vi "Insert Stop Message.vi"(8 "error in (no error)":errorcluster, 11 "TimeStamper in":refnum<class "TimeStamper.lvclass">) -> (0 "error out":errorcluster, 3 "TimeStamper out":refnum<class "TimeStamper.lvclass">)   [LabVIEW 2014, in "TimeStamper.lvclass"]
uses:
  TimeStamper.lvclass
  Database/SessionPrimary.ctl
  AcquistionObject/AcquistionObject.lvclass
panel:
  out "resulting string":string
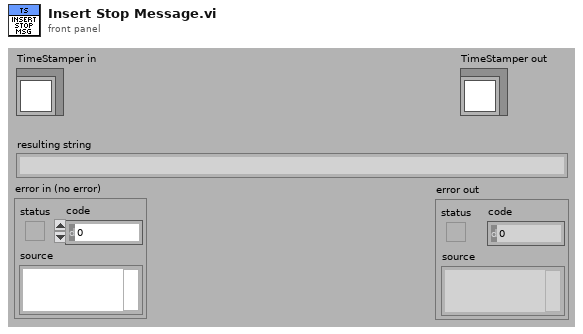
[diagram p1: front panel]
types:
  T1 = typedef "SessionPrimary.ctl" = cluster{"setup":u8, "subject_id":i32, "session_start_time":dbl}
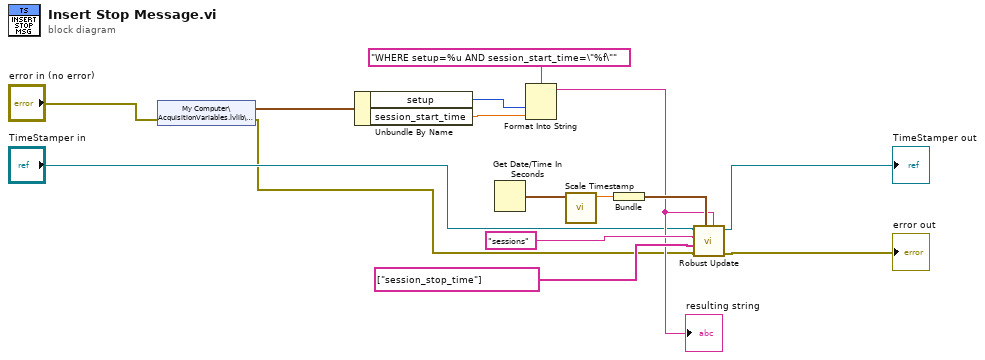
[diagram p0: block diagram]
diagram:
  n1 = shared-variable "My Computer\\AcquisitionVariables.lvlib\\SessionPK"(error in="error in (no error)") -> (w13:T1, error out=w2:errorcluster)
  n2 = Unbundle By Name(w13) -> ("setup"=w11:u8, "session_start_time"=w10:dbl)
  n3 = Get Date/Time In Seconds() -> (seconds since 1Jan1904=w14:timestamp)
  n4 = Format Into String(format string="WHERE setup=%u AND session_start_time=\"%f\"", w11, w10) -> (resulting string=w4:string)  [unwired: 2 in, 1 out]
  "resulting string" <- w4
  n5 = call "Scale Timestamp.vi"("Time Stamp"=w14) -> ("Scaled timestamp"=w9:dbl)  [unwired: 10 in]
  n6 = Bundle("Scaled timestamp"=w9) -> (w5:cluster{"Scaled timestamp":dbl})  [unwired: 1 in]
  n7 = call "Robust Update.vi"("condition"=w4, "data"=w5, "error in (no error)"=w2, "columns"=string[] ["session_stop_time"], "table"="sessions", "AcquistionObject.lvclass"="TimeStamper in") -> ("error out"=→"error out":errorcluster, "AcquistionObject out"=→"TimeStamper out":refnum<class "TimeStamper.lvclass">)  [unwired: 4 in]
